vi "Get OnOff.Act.vi"(8 "error in":errorcluster, 11 "Device Cluster.lvclass in":refnum<class "Device Cluster.lvclass">) -> (0 "error out":errorcluster, 2 "OnOff.ACT":bool, 3 "Device Cluster.lvclass out":refnum<class "Device Cluster.lvclass">)   [LabVIEW 2023, in "Device Cluster.lvclass"]
uses:
  Device Cluster.lvclass
  Device Cluster.lvclass/Device Cluster.ctl
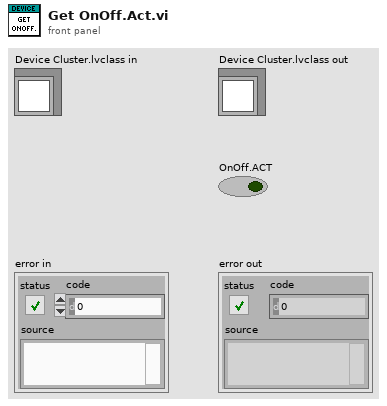
[diagram p1: front panel]
types:
  T1 = typedef "Cluster.lvclass/Consumer Control.ctl" = cluster{"OnOff.ACT":bool, "ErrorAcknowledge.ACT":bool}
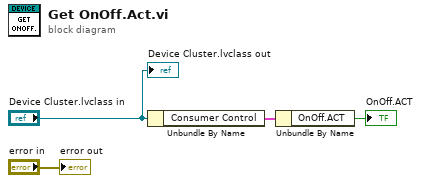
[diagram p0: block diagram]
diagram:
  n1 = Unbundle By Name("Device Cluster.lvclass in") -> ("Consumer Control"=w3:T1)
  n2 = Unbundle By Name(w3) -> ("OnOff.ACT"=→"OnOff.ACT":bool)
  "Device Cluster.lvclass out" <- "Device Cluster.lvclass in"
  "error out" <- "error in"
